vi "Decimate.vi"(11 "ExpFitter in":refnum<class "ExpFitter.lvclass">) -> (2 "data valid":bool, 3 "ExpFitter out":refnum<class "ExpFitter.lvclass">)   [LabVIEW 2019, in "ExpFitter.lvclass"]
uses:
  ExpFitter.lvclass
  ExpFitter.lvclass/ExpFitter.ctl
  <vilib>/Analysis/2dsp.llb/Decimate (single shot, DBL).vi
  <vilib>/Analysis/NI_AALPro.lvlib
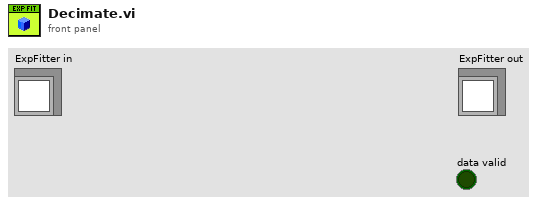
[diagram p1: front panel]
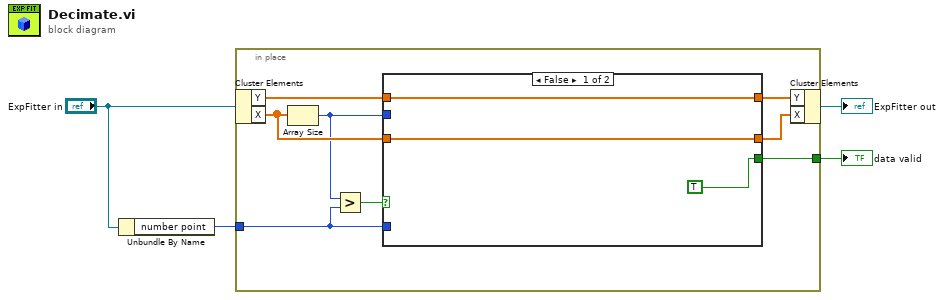
[diagram p0: block diagram]
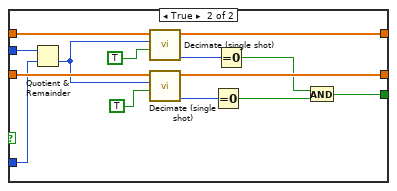
[diagram p2: hidden frame]
diagram:
  n1 = Unbundle By Name("ExpFitter in") -> ("number point"=w2:i32)
  n2 = in-place {
    in-place-border: w2 -> [w6]
    in-place-border: [w5] -> w1
    n3 = in-place-cluster #1("ExpFitter in") -> ("Y"=w10:dbl[], "X"=w8:dbl[])
    n4 = Array Size(array=w8) -> (size(s)=w7:i32)
    n5 = Greater?(x=w7, y=w6) -> (0:w12:bool)
    n6 = case shown="False" w12 {
      tunnel: [w15 w27] -> w11
      tunnel: w10 -> [w15 w28]
      tunnel: w8 -> [w14 w25]
      tunnel: [w14 w24] -> w9
      tunnel: w7 -> [_ w23]
      tunnel: w6 -> [_ w22]
      tunnel: [TRUE w16] -> w5
      frame False {
      }
      frame True {
        n7 = Quotient & Remainder(x=w23, y=w22) -> (floor(x/y)=w21:i32)  [unwired: 1 out]
        n8 = call-poly <vilib>:"Decimate (single shot).vi"("averaging"=TRUE, "decimating factor"=w21, "X"=w28) -> ("error"=w19:i32, "Decimated Array"=w27:dbl[])  [unwired: 7 in]
        n9 = call-poly <vilib>:"Decimate (single shot).vi"("averaging"=TRUE, "decimating factor"=w21, "X"=w25) -> ("error"=w20:i32, "Decimated Array"=w24:dbl[])  [unwired: 7 in]
        n10 = Equal To 0?(x=w20) -> (x = 0?=w17:bool)
        n11 = Equal To 0?(x=w19) -> (x = 0?=w18:bool)
        n12 = And(x=w18, y=w17) -> (x .and. y?=w16:bool)
      }
    }
    n13 = in-place-cluster #1("Y"=w11, "X"=w9) -> (→"ExpFitter out":refnum<class "ExpFitter.lvclass">)
  }
  "data valid" <- w1
